vi "find zero crossings detector.vi"(0 "display queues":T2, 5 "slope":bool=TRUE, 7 "hysteresis":dbl=0.05 format="%#_13g", 11 "error in (no error)":errorcluster) -> (2 "crossing stats":T1, 3 "period":dbl, 4 "recent crossing":dbl, 6 "prev crossing":dbl, 8 "crossing-2":dbl, 10 "new crossing":bool, 14 "number of crossings":i32, 15 "error out":errorcluster)   [LabVIEW 2017]
uses:
  typedefs/queue cluster.ctl
  typedefs/reading queue.ctl
  typedefs/reading.ctl
  typedefs/readingType.ctl
  typedefs/reading1.ctl
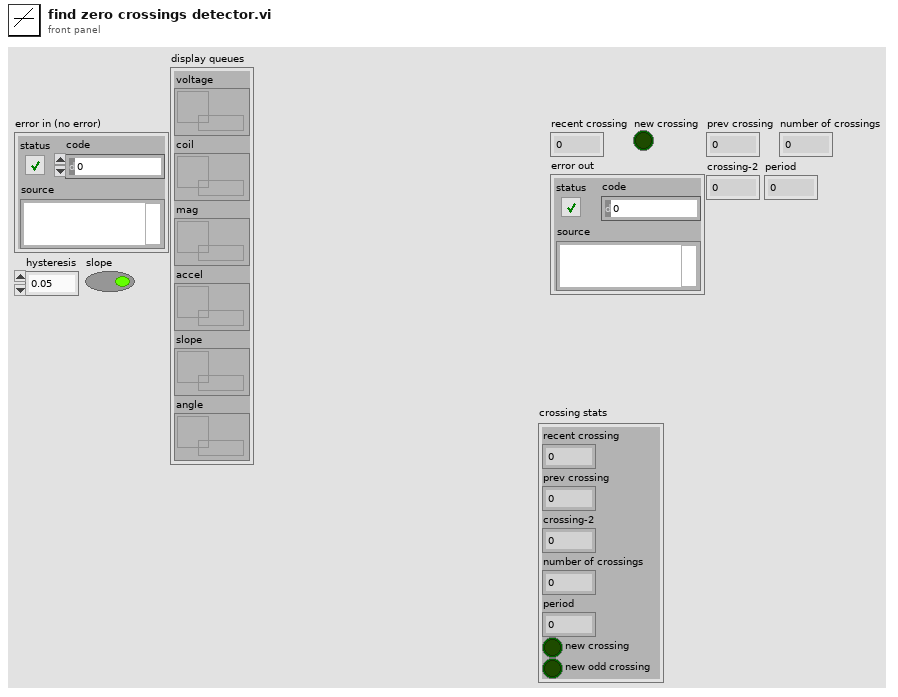
[diagram p1: front panel]
types:
  T1 = cluster{"recent crossing":dbl, "prev crossing":dbl, "crossing-2":dbl, "number of crossings":i32, "period":dbl, "new crossing":bool, "new odd crossing":bool}
  T2 = typedef "queue cluster.ctl" = cluster{"voltage":T3, "coil":T3, "mag":T3, "accel":T3, "slope":refnum<queue>, "angle":refnum<queue>}
  T3 = typedef "reading queue.ctl" = refnum<queue>
  T4 = typedef "reading.ctl" = cluster{"reading type":T5, "time":fxp<+,48,48>, "x":sgl, "y":sgl, "z":sgl, "XSUM":u8}
  T5 = typedef "readingType.ctl" = enum8{"SYNC", "DETVAL", "COILI", "MAGVEC", "ACCVEC"}
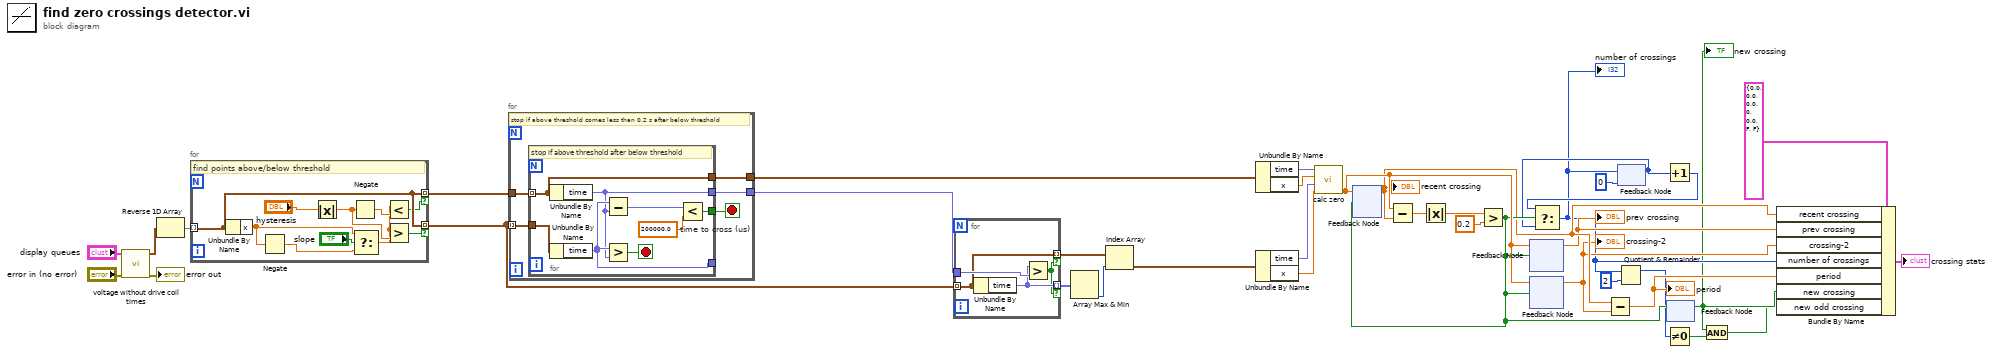
[diagram p0: block diagram]
diagram:
  n1 = call "voltage without drive coil times.vi"("error in (no error)"="error in (no error)", "display queues"="display queues") -> ("error out"=→"error out":errorcluster, "voltage_no_coil"=w20:T4[])  [unwired: 7 in, 1 out]
  n2 = Reverse 1D Array(array=w20) -> (reversed array=w19:T4[])
  n3 = for {
    tunnel: w19 -> [w39] mode=indexing
    tunnel: [w39] -> w33 mode=indexing if=w43
    tunnel: [w39] -> w37 mode=indexing if=w38
    # "find points above/below threshold"
    n4 = Unbundle By Name(w39) -> ("x"=w46:sgl)
    n5 = Negate(x=w46) -> (-x=w45:sgl)
    n6 = Absolute Value(x="hysteresis") -> (abs(x)=w42:dbl)
    n7 = Negate(x=w42) -> (-x=w41:dbl)
    n8 = Select(t=w46, s="slope", f=w45) -> (s? t:f=w40:sgl)
    n9 = Less?(x=w40, y=w41) -> (x < y?=w38:bool)
    n10 = Greater?(x=w40, y=w42) -> (0:w43:bool)
  }
  n11 = for {
    tunnel: w33 -> [w52] mode=indexing
    tunnel: w37 -> [w51]
    tunnel: [w49] -> w32
    tunnel: [w48] -> w28
    stop <- w50 stop-if-true
    # "stop if above threshold comes less than 0.2 s after below threshold"
    n12 = for {
      tunnel: w52 -> [w60]
      tunnel: w51 -> [w53] mode=indexing
      tunnel: [w56] -> w50
      tunnel: [w55] -> _
      tunnel: [w54] -> w49
      tunnel: [w53] -> w48
      stop <- w59 stop-if-true
      w57 = 200000.0  # time to cross (us)
      # "stop if above threshold after below threshold"
      n13 = Unbundle By Name(w53) -> ("time"=w54:fxp<+,48,48>)
      n14 = Unbundle By Name(w60) -> ("time"=w55:fxp<+,48,48>)
      n15 = Subtract(x=w55, y=w54) -> (x-y=w58:fxp<+/-,49,49>)
      n16 = Greater?(x=w55, y=w54) -> (0:w59:bool)
      n17 = Less?(x=w58, y=w57) -> (x < y?=w56:bool)
    }
  }
  n18 = for {
    tunnel: w33 -> [w63] mode=indexing
    tunnel: w32 -> [w64]
    tunnel: [w63] -> w30 mode=indexing if=w61
    tunnel: [w62] -> w31 mode=indexing if=w61
    n19 = Unbundle By Name(w63) -> ("time"=w62:fxp<+,48,48>)
    n20 = Greater?(x=w62, y=w64) -> (0:w61:bool)
  }
  n21 = Array Max & Min(array=w31) -> (min index (indices)=w29:i32)  [unwired: 3 out]
  n22 = Index Array(array=w30, index=w29) -> (element=w27:T4)
  n23 = Unbundle By Name(w28) -> ("time"=w26:fxp<+,48,48>, "x"=w25:sgl)
  n24 = Unbundle By Name(w27) -> ("time"=w24:fxp<+,48,48>, "x"=w23:sgl)
  n25 = call "calc zero.vi"("x2"=w23, "t2 (us)"=w24, "x1"=w25, "t1 (us)"=w26) -> ("tcross (s)"=w22:dbl)  [unwired: 7 in]
  n26 = feedback #1() -> (w12:dbl)  [unwired: 1 in]
  "recent crossing" <- w12
  n27 = Subtract(x=w22, y=w12) -> (x-y=w36:dbl)
  n28 = Absolute Value(x=w36) -> (abs(x)=w35:dbl)
  n29 = Greater?(x=w35, y=0.2) -> (0:w14:bool)
  n30 = feedback-in #1(w22, w14) -> ()
  n31 = feedback-in #2(w22, w14) -> ()
  n32 = feedback #2() -> (w11:dbl)  [unwired: 1 in]
  "prev crossing" <- w11
  n33 = feedback #3() -> (w10:dbl)  [unwired: 1 in]
  "crossing-2" <- w10
  n34 = feedback-in #3(w22, w14) -> ()
  n35 = Subtract(x=w12, y=w10) -> (x-y=w9:dbl)
  "period" <- w9
  n36 = feedback #4(0) -> (w13:i32)
  n37 = Increment(x=w13) -> (x+1=w16:i32)
  n38 = Select(t=w16, s=w14, f=w13) -> (s? t:f=w6:i32)
  "number of crossings" <- w6
  n39 = feedback-in #4(w6) -> ()
  n40 = Quotient & Remainder(x=w6, y=2) -> (x-y*floor(x/y)=w4:i32)  [unwired: 1 out]
  n41 = Not Equal To 0?(x=w4) -> (x != 0?=w3:bool)
  n42 = feedback-in #5(w14) -> ()
  n43 = feedback #5() -> (w2:bool)  [unwired: 1 in]
  "new crossing" <- w2
  n44 = And(x=w2, y=w3) -> (x .and. y?=w1:bool)
  n45 = Bundle By Name(cluster=T1 {"recent crossing"=0.0, "prev crossing"=0.0, "crossing-2"=0.0, "number of crossings"=0, "period"=0.0, "new crossing"=FALSE, "new odd crossing"=FALSE} ("crossing stats"), "recent crossing"=w12, "prev crossing"=w11, "crossing-2"=w10, "number of crossings"=w6, "period"=w9, "new crossing"=w2, "new odd crossing"=w1) -> (→"crossing stats":T1)
